vi "Build analog waveform.vi"(0 "System no.":i32=1 min=1 step=1, 1 "Index of axis":i32 min=0 step=1, 2 "Start voltage":dbl format="%.8f", 3 "Target voltage":dbl format="%.8f", 5 "error in":errorcluster) -> (14 "Waveform":waveform(dbl), 15 "T (s)":dbl, 16 "Start = Target?":bool, 19 "error out":errorcluster)   [LabVIEW 2020]
doc: "This vi returns a waveform calculated by start and target voltage for the given axis.\n\nValid for Analog Systems."
uses:
  Global Analog.vi
panel:
  out "HyperBit Bits":dbl
  out "N":dbl
  # "This vi returns a waveform calculated by start and target voltage for the given axis."
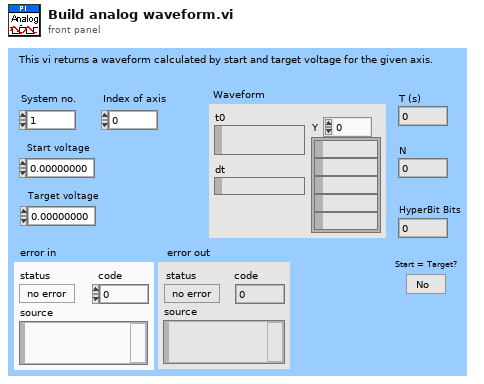
[diagram p1: front panel]
types:
  T1 = cluster{"Conversion factor":dbl[], "Velocity":dbl[], "Velocity control mode":bool, "AO.Resolution":dbl, "Lower voltage limit (V)":dbl, "Upper voltage limit (V)":dbl, "AO_WF_T (s)":dbl, "AI Sample Rate":dbl, "AI Samples/Channel":i32, "Hyperbit":bool, "Offset (V)":dbl[], "Hyperbit StayOnPos":bool, "Gain (V)":dbl[], "Bit rate (Hz)":dbl, "PWM rate (Hz)":dbl, "HyperBit Password":string, "AO.MaxRate":dbl, "Conversion offset":dbl[]}[]
  T2 = cluster{"Conversion factor":dbl[], "Velocity":dbl[], "Velocity control mode":bool, "AO.Resolution":dbl, "Lower voltage limit (V)":dbl, "Upper voltage limit (V)":dbl, "AO_WF_T (s)":dbl, "AI Sample Rate":dbl, "AI Samples/Channel":i32, "Hyperbit":bool, "Offset (V)":dbl[], "Hyperbit StayOnPos":bool, "Gain (V)":dbl[], "Bit rate (Hz)":dbl, "PWM rate (Hz)":dbl, "HyperBit Password":string, "AO.MaxRate":dbl, "Conversion offset":dbl[]}
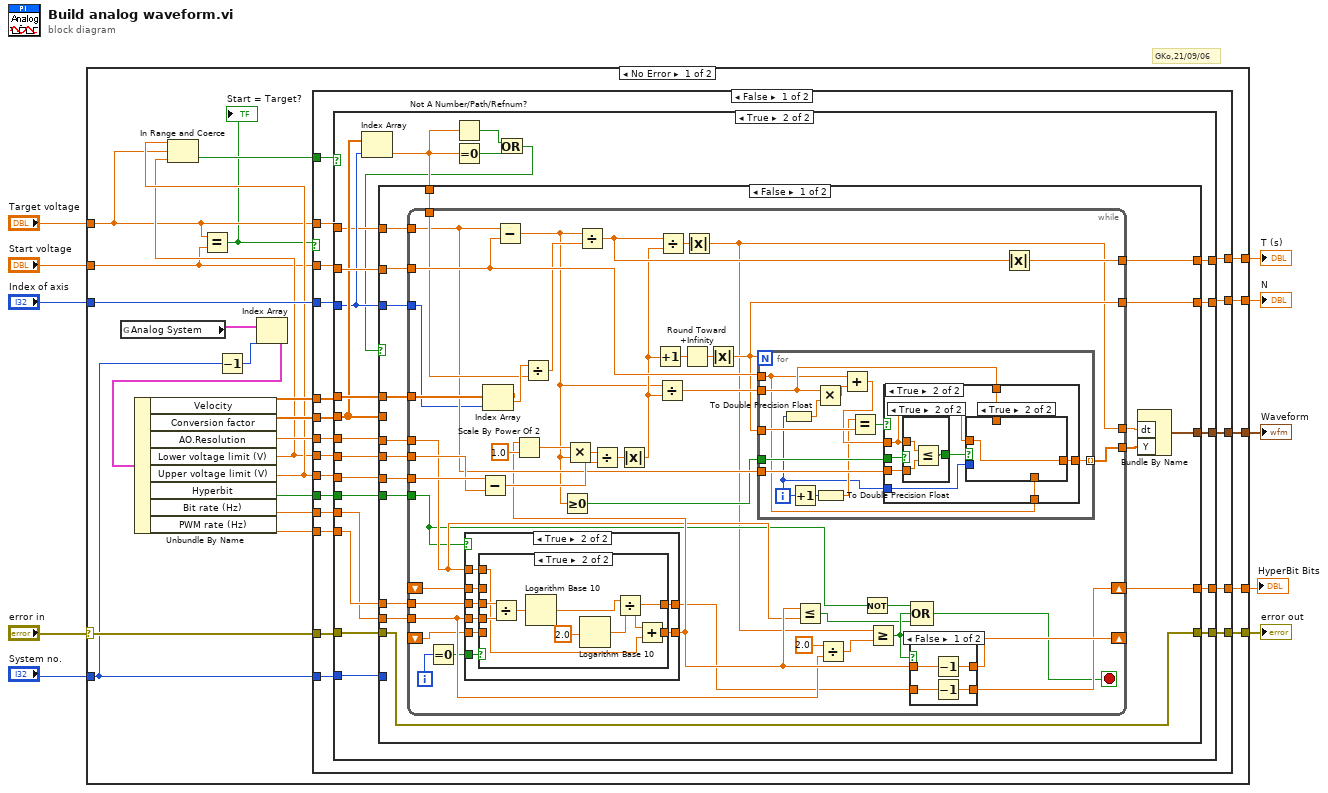
[diagram p0: block diagram]
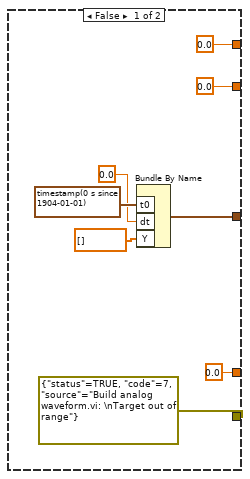
[diagram p2: hidden frame]
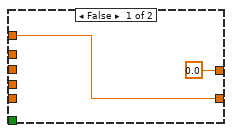
[diagram p4: hidden frame]
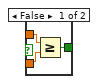
[diagram p7: hidden frame]
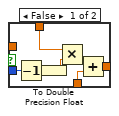
[diagram p8: hidden frame]
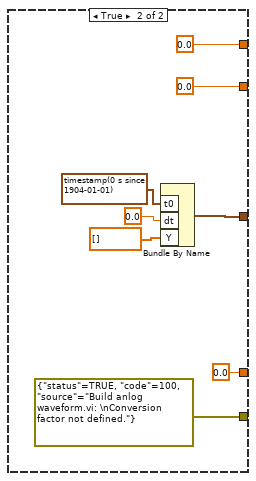
[diagram p9: hidden frame]
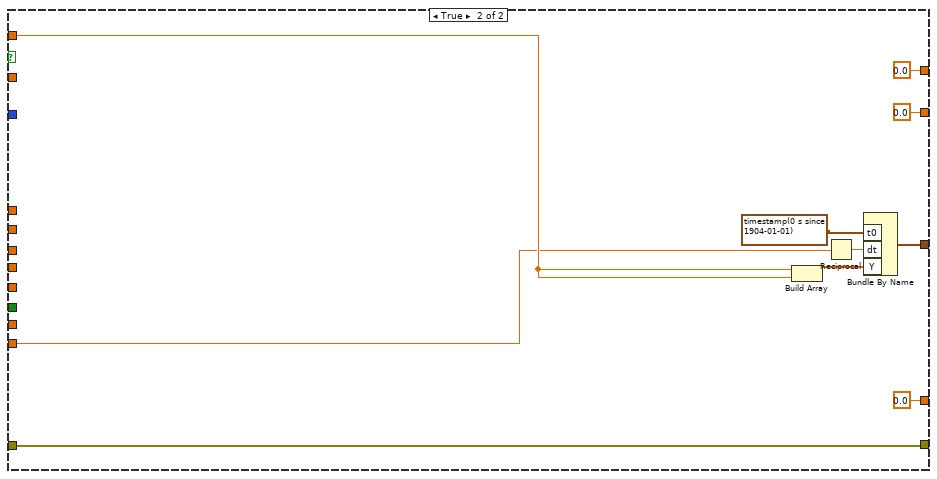
[diagram p10: hidden frame]
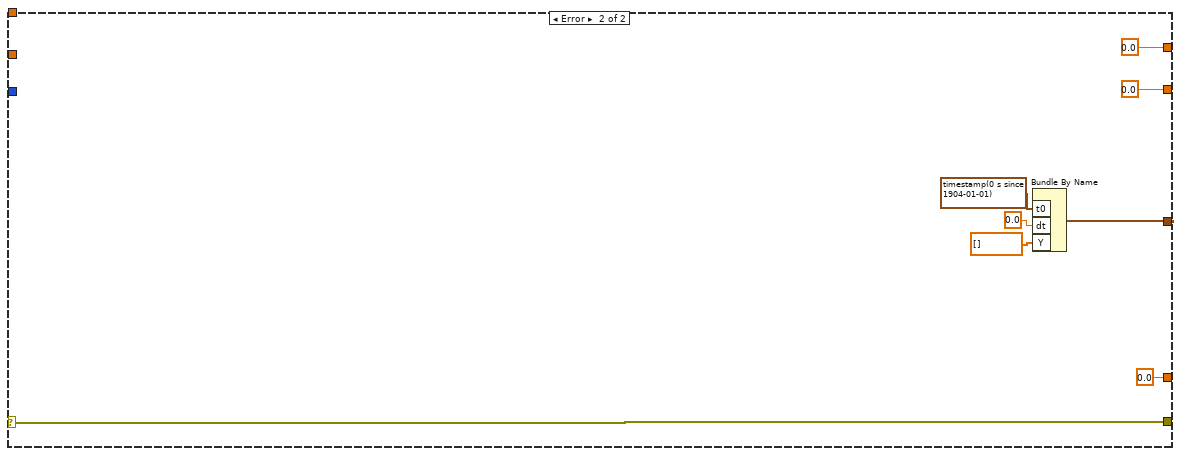
[diagram p11: hidden frame]
diagram:
  # "GKo,21/09/06"
  n1 = case shown="No Error" "error in" {
    selector: "error in" -> [w26 w233]
    tunnel: [w25 w233] -> w9
    tunnel: "System no." -> [w20 _]
    tunnel: "Index of axis" -> [w27 _]
    tunnel: "Target voltage" -> [w14 _]
    tunnel: "Start voltage" -> [w13 _]
    tunnel: [w24 w231] -> w4
    tunnel: [w19 0.0] -> w3
    tunnel: [w18 0.0] -> w2
    tunnel: [w11 0.0] -> w1
    frame No Error {
      n2 = global read "Global Analog.vi" "Analog System"() -> (w33:T1)
      n3 = Equal?(x=w14, y=w13) -> (x = y?=w12:bool)
      "Start = Target?" <- w12
      n4 = Decrement(x=w20) -> (x-1=w32:i32)
      n5 = Index Array(array=w33, index=w32) -> (element=w31:T2)
      n6 = Unbundle By Name(w31) -> ("Velocity"=w30:dbl[], "Conversion factor"=w28:dbl[], "AO.Resolution"=w29:dbl, "Lower voltage limit (V)"=w22:dbl, "Upper voltage limit (V)"=w23:dbl, "Hyperbit"=w17:bool, "Bit rate (Hz)"=w15:dbl, "PWM rate (Hz)"=w16:dbl)
      n7 = In Range and Coerce(upper limit=w23, x=w14, lower limit=w22) -> (In Range?=w21:bool)  [unwired: 1 out]
      n8 = case shown="False" w12 {
        tunnel: w30 -> [w52 _]
        tunnel: w29 -> [w51 _]
        tunnel: w28 -> [w50 _]
        tunnel: w27 -> [w49 _]
        tunnel: w26 -> [w48 w221]
        tunnel: [w47 w221] -> w25
        tunnel: [w46 w222] -> w24
        tunnel: w23 -> [w45 _]
        tunnel: w22 -> [w44 _]
        tunnel: w21 -> [w43 _]
        tunnel: w20 -> [w42 _]
        tunnel: [w41 0.0] -> w19
        tunnel: [w40 0.0] -> w18
        tunnel: w17 -> [w39 _]
        tunnel: w16 -> [w38 w216]
        tunnel: w15 -> [w37 _]
        tunnel: w14 -> [w36 w218]
        tunnel: w13 -> [w35 _]
        tunnel: [w34 0.0] -> w11
        frame False {
          n9 = case shown="True" w43 {
            tunnel: w52 -> [_ w82]
            tunnel: w51 -> [_ w81]
            tunnel: w35 -> [_ w80]
            tunnel: w50 -> [_ w79]
            tunnel: w49 -> [_ w78]
            tunnel: w48 -> [_ w69]
            tunnel: [errorcluster {"status"=TRUE, "code"=7, "source"="Build analog waveform.vi: \nTarget out of range"} ("error out") w70] -> w47
            tunnel: [w59 w74] -> w46
            tunnel: w36 -> [_ w73]
            tunnel: w45 -> [_ w72]
            tunnel: w44 -> [_ w68]
            tunnel: w42 -> [_ w67]
            tunnel: [0.0 w66] -> w41
            tunnel: [0.0 w65] -> w40
            tunnel: w39 -> [_ w64]
            tunnel: w38 -> [_ w63]
            tunnel: w37 -> [_ w62]
            tunnel: [0.0 w61] -> w34
            frame False {
              n10 = Bundle By Name("t0"=timestamp(0 s since 1904-01-01), "dt"=0.0, "Y"=dbl[] []) -> (w59:waveform(dbl))  [unwired: 1 out]
            }
            frame True {
              n11 = Index Array(array=w79, index=w78) -> (element=w75:dbl)
              n12 = Not A Number/Path/Refnum?(number/path/refnum=w75) -> (NaN/Path/Refnum?=w77:bool)
              n13 = Equal To 0?(x=w75) -> (x = 0?=w76:bool)
              n14 = Or(x=w77, y=w76) -> (x .or. y?=w71:bool)
              n15 = case shown="False" w71 {
                tunnel: w82 -> [w100 _]
                tunnel: w81 -> [w87 _]
                tunnel: w80 -> [w99 _]
                tunnel: w79 -> [_ _]
                tunnel: w78 -> [w92 _]
                tunnel: w75 -> [w98 _]
                tunnel: [w96 w212] -> w74
                tunnel: w73 -> [w93 _]
                tunnel: w72 -> [w95 _]
                tunnel: w68 -> [w94 _]
                tunnel: [w84 errorcluster {"status"=TRUE, "code"=100, "source"="Build anlog waveform.vi: \nConversion factor not defined."} ("error out")] -> w70
                tunnel: w69 -> [w84 _]
                tunnel: w67 -> [_ _]
                tunnel: [w91 0.0] -> w66
                tunnel: [w90 0.0] -> w65
                tunnel: w64 -> [w88 _]
                tunnel: w63 -> [w86 _]
                tunnel: w62 -> [w85 _]
                tunnel: [w83 0.0] -> w61
                frame False {
                  n16 = while {
                    tunnel: w100 -> [w144]
                    tunnel: w99 -> [w141]
                    tunnel: w98 -> [w134]
                    tunnel: [w102] -> w97
                    tunnel: w95 -> [w128]
                    tunnel: w94 -> [w127]
                    tunnel: w93 -> [w126]
                    tunnel: w92 -> [w123]
                    tunnel: [w122] -> w91
                    tunnel: [w121] -> w90
                    tunnel: [w101] -> w89
                    tunnel: w88 -> [w104]
                    tunnel: w87 -> [w111]
                    tunnel: w86 -> [w120]
                    tunnel: w85 -> [w112]
                    shift-right: [w115] -> _
                    shift-left: _ -> [w108]
                    shift-right: [w106] -> w83
                    shift-left: _ -> [w105]
                    i -> [w110]
                    stop <- w103 stop-if-true
                    n17 = Equal To 0?(x=w110) -> (x = 0?=w109:bool)
                    n18 = case shown="True" w104 {
                      tunnel: w111 -> [w152 w158]
                      tunnel: w120 -> [_ w160]
                      tunnel: w112 -> [_ w159]
                      tunnel: [w152 w157] -> w113
                      tunnel: w109 -> [_ w156]
                      tunnel: w108 -> [_ w155]
                      tunnel: [0.0 w154] -> w107
                      tunnel: w105 -> [_ w153]
                      frame False {
                      }
                      frame True {
                        n19 = case shown="True" w156 {
                          tunnel: w160 -> [_ w171]
                          tunnel: w159 -> [_ w170]
                          tunnel: w158 -> [_ w165]
                          tunnel: [w162 w164] -> w157
                          tunnel: w155 -> [w162 _]
                          tunnel: [w161 w163] -> w154
                          tunnel: w153 -> [w161 _]
                          frame False {
                          }
                          frame True {
                            n20 = Divide(x=w171, y=w170) -> (x/y=w169:dbl)
                            n21 = Logarithm Base 10(1:w169) -> (0:w167:dbl)
                            n22 = Logarithm Base 10(1:2.0 ("x")) -> (0:w166:dbl)
                            n23 = Divide(x=w167, y=w166) -> (x/y=w163:dbl)
                            n24 = Add(x=w163, y=w165) -> (x+y=w164:dbl)
                          }
                        }
                      }
                    }
                    n25 = Subtract(x=w128, y=w127) -> (x-y=w138:dbl)
                    n26 = Index Array(array=w144, index=w123) -> (element=w135:dbl)
                    n27 = Subtract(x=w126, y=w141) -> (x-y=w125:dbl)
                    n28 = Scale By Power Of 2(n=w113, x=1.0) -> (x*2^n=w140:dbl)
                    n29 = Divide(x=w135, y=w134) -> (x/y=w136:dbl)
                    n30 = Greater Or Equal To 0?(x=w125) -> (x >= 0?=w124:bool)
                    n31 = Multiply(x=w140, y=w125) -> (x*y=w139:dbl)
                    n32 = Divide(x=w125, y=w136) -> (x/y=w143:dbl)
                    n33 = Divide(x=w139, y=w138) -> (x/y=w131:dbl)
                    n34 = Absolute Value(x=w131) -> (abs(x)=w130:dbl)
                    n35 = Increment(x=w130) -> (x+1=w133:dbl)
                    n36 = Divide(x=w125, y=w130) -> (x/y=w137:dbl)
                    n37 = Divide(x=w143, y=w130) -> (x/y=w129:dbl)
                    n38 = Round Toward +Infinity(x=w133) -> (ceil(x): smallest int >= x=w132:dbl)
                    n39 = Absolute Value(x=w129) -> (abs(x)=w102:dbl)
                    n40 = Absolute Value(x=w132) -> (abs(x)=w121:dbl)
                    n41 = for {
                      N: w121 -> [_]
                      tunnel: w141 -> [w172]
                      tunnel: [w179] -> w101 mode=indexing
                      tunnel: w137 -> [w173]
                      tunnel: w121 -> [w182]
                      tunnel: w126 -> [w181]
                      tunnel: w124 -> [w177]
                      i -> [w174]
                      n42 = To Double Precision Float(number=w174) -> (double precision float=w176:dbl)
                      n43 = Increment(x=w174) -> (x+1=w183:i32)
                      n44 = Multiply(x=w173, y=w176) -> (x*y=w184:dbl)
                      n45 = To Double Precision Float(number=w183) -> (double precision float=w175:dbl)
                      n46 = Add(x=w172, y=w184) -> (x+y=w180:dbl)
                      n47 = Equal?(x=w175, y=w182) -> (x = y?=w178:bool)
                      n48 = case shown="True" w178 {
                        tunnel: w180 -> [w185 w191]
                        tunnel: w181 -> [_ w189]
                        tunnel: [w185 w193] -> w179
                        tunnel: w177 -> [_ w192]
                        tunnel: w174 -> [_ w188]
                        tunnel: w173 -> [_ w187]
                        tunnel: w172 -> [_ w186]
                        frame False {
                        }
                        frame True {
                          n49 = case shown="True" w192 {
                            tunnel: w191 -> [w195 w199]
                            tunnel: w189 -> [w194 w197]
                            tunnel: [w196 w198] -> w190
                            frame False {
                              n50 = Greater Or Equal?(x=w195, y=w194) -> (x >= y?=w196:bool)
                            }
                            frame True {
                              n51 = Less Or Equal?(x=w199, y=w197) -> (x <= y?=w198:bool)
                            }
                          }
                          n52 = case shown="True" w190 {
                            tunnel: [w200 w207] -> w193
                            tunnel: w191 -> [_ w207]
                            tunnel: w188 -> [w206 _]
                            tunnel: w187 -> [w203 _]
                            tunnel: w186 -> [w201 _]
                            frame False {
                              n53 = Decrement(x=w206) -> (x-1=w205:i32)
                              n54 = To Double Precision Float(number=w205) -> (double precision float=w204:dbl)
                              n55 = Multiply(x=w203, y=w204) -> (x*y=w202:dbl)
                              n56 = Add(x=w202, y=w201) -> (x+y=w200:dbl)
                            }
                            frame True {
                            }
                          }
                        }
                      }
                    }
                    n57 = Less Or Equal?(x=w113, y=w111) -> (x <= y?=w114:bool)
                    n58 = Divide(x=2.0, y=w112) -> (x/y=w117:dbl)
                    n59 = Not(x=w104) -> (.not. x?=w119:bool)
                    n60 = Greater Or Equal?(x=w102, y=w117) -> (x >= y?=w116:bool)
                    n61 = case shown="False" w116 {
                      tunnel: w113 -> [w148 w150]
                      tunnel: [w147 w150] -> w115
                      tunnel: [w146 w149] -> w106
                      tunnel: w107 -> [w145 w149]
                      frame False {
                        n62 = Decrement(x=w148) -> (x-1=w147:dbl)
                        n63 = Decrement(x=w145) -> (x-1=w146:dbl)
                      }
                      frame True {
                      }
                    }
                    n64 = Compound Arithmetic op=OR(w119, w116, w114) -> (w103:bool)
                    n65 = Absolute Value(x=w143) -> (abs(x)=w122:dbl)
                  }
                  n66 = Bundle By Name("dt"=w97, "Y"=w89) -> (w96:waveform(dbl))  [unwired: 1 out]
                }
                frame True {
                  n67 = Bundle By Name("t0"=timestamp(0 s since 1904-01-01), "dt"=0.0, "Y"=dbl[] []) -> (w212:waveform(dbl))  [unwired: 1 out]
                }
              }
            }
          }
        }
        frame True {
          n68 = Build Array(w218, w218) -> (w219:dbl[])
          n69 = Reciprocal(x=w216) -> (1/x=w217:dbl)
          n70 = Bundle By Name("t0"=timestamp(0 s since 1904-01-01), "dt"=w217, "Y"=w219) -> (w222:waveform(dbl))  [unwired: 1 out]
        }
      }
    }
    frame Error {
      n71 = Bundle By Name("t0"=timestamp(0 s since 1904-01-01), "dt"=0.0, "Y"=dbl[] []) -> (w231:waveform(dbl))  [unwired: 1 out]
    }
  }
  "error out" <- w9
  "Waveform" <- w4
  "T (s)" <- w3
  "N" <- w2
  "HyperBit Bits" <- w1
